vi "Close ConvBox Handler.vi"(8 "error in (no error)":errorcluster, 11 "Listener in":refnum<class "Listener.lvclass">) -> (0 "error out":errorcluster, 3 "Listener out":refnum<class "Listener.lvclass">)   [LabVIEW 2023, in "Listener.lvclass"]
uses:
  Listener.lvclass
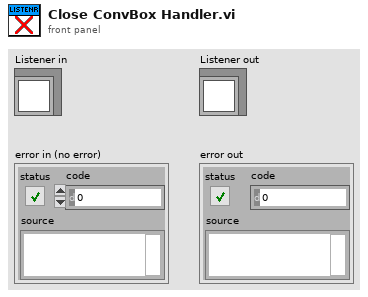
[diagram p1: front panel]
types:
  T1 = typedef "Listener.lvclass/RS-xxx To GPIB ConvBox Data Structure.ctl" = cluster{"Data":string, "Command Messages Read":string[], "Address":string, "Data Length":u32}
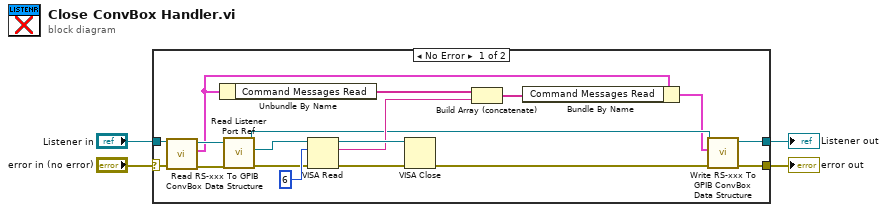
[diagram p0: block diagram]
diagram:
  n1 = case shown="No Error" "error in (no error)" {
    selector: "error in (no error)" -> [w16 w24]
    tunnel: [w10 w24] -> w3
    tunnel: "Listener in" -> [w17 w23]
    tunnel: [w9 w23] -> w1
    frame No Error {
      n2 = call-dynamic "Read RS-xxx To GPIB ConvBox Data Structure.vi"("error in (no error)"=w16, "Listener in"=w17) -> ("error out"=w15:errorcluster, "RS-xxx To GPIB ConvBox Data Structure"=w7:T1, "Listener out"=w14:refnum<class "Listener.lvclass">)  [unwired: 7 in]
      n3 = Unbundle By Name(w7) -> ("Command Messages Read"=w13:string[])
      n4 = call "Read Listener Port Ref.vi"("error in (no error)"=w15, "Listener in"=w14) -> ("error out"=w19:errorcluster, "Listener Port Ref"=w18:refnum<visa-resource-name>, "Listener out"=w8:refnum<class "Listener.lvclass">)  [unwired: 7 in]
      n5 = VISA Read(VISA resource name=w18, byte count=u32 6, error in (no error)=w19) -> (VISA resource name out=w21:refnum<visa-resource-name>, read buffer=w12:string, error out=w20:errorcluster)  [unwired: 1 out]
      n6 = VISA Close(VISA resource name=w21, error in (no error)=w20) -> (error out=w11:errorcluster)
      n7 = Build Array (concatenate)(w13, w12) -> (w6:string[])
      n8 = Bundle By Name(cluster=w7, "Command Messages Read"=w6) -> (w5:T1)
      n9 = call-dynamic "Write RS-xxx To GPIB ConvBox Data Structure.vi"("error in (no error)"=w11, "RS-xxx To GPIB ConvBox Data Structure"=w5, "Listener in"=w8) -> ("error out"=w10:errorcluster, "Listener out"=w9:refnum<class "Listener.lvclass">)  [unwired: 7 in]
    }
    frame Error {
    }
  }
  "error out" <- w3
  "Listener out" <- w1
